vi "get_some_points.vi"(0 "Override":T3, 2 "Stimulus":T1={"Type"=enum."Off", "Phase"=0.0, "Amplitude"=[0.0, 0.0, 0.0, 0.0, 0.0, 0.0], "Injection point"=enum."Total pose", "Closed loop"=TRUE, "Offset"=[0.0, 0.0, 0.0, 0.0, 0.0, 0.0], "Tip -> world"=FALSE, "Frequency"=0.0, "Length"=0.0} {"Length" min=0.0 max=100.0 step=100.0 format="%#_4p"; "Frequency" min=0.0 step=100.0 format="%#_4g"; "Offset" format="%#_3p"; "Amplitude" format="%#_3p"; "Phase" min=-180.0 max=360.0 step=100.0 format="%#.2f"}, 3 "Trace length":dbl=1.0, 5 "Axis names":string[](array[string])=["X", "Y", "Z", "Rx", "Ry", "Rz"], 7 "Sequence":dbl[][](array[numeric]), 11 "error in":errorcluster, 12 "Position mode":enum16{"Absolute axis", "Relative axis", "Pose"}(ring), 14 "Decimate":i32=-1) -> (6 "Decimated trace":sgl[][][][](array[numeric]) format="%#_5g", 15 "error out":errorcluster)   [LabVIEW 2013]
uses:
  ui_override_opts.ctl
  stimulus.ctl
  injection_point.ctl
panel:
  # "This VI uses the motion interface to move the stage to a sequence of points.  At each point it triggers a trace cycle and captures the trace data.  Use with ui_override.vi and single_trigger_setup.vi."
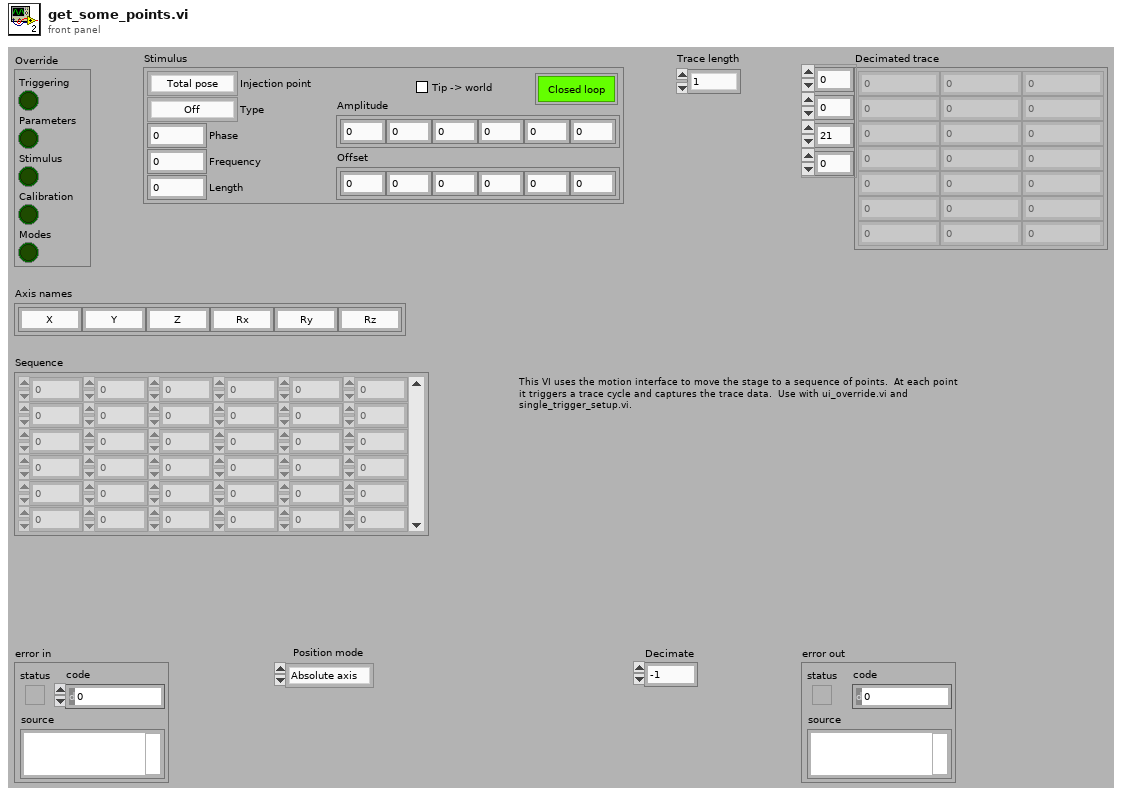
[diagram p1: front panel]
types:
  T1 = typedef "stimulus.ctl" = cluster{"Type":enum16{"Off", "Step", "Sine", "Triangle", "Arbitrary"}, "Phase":dbl, "Amplitude":sgl[], "Injection point":T2, "Closed loop":bool, "Offset":sgl[], "Tip -> world":bool, "Frequency":dbl, "Length":dbl}
  T2 = typedef "injection_point.ctl" = enum16{"Total pose", "V limiter", "Goal ", "Link position", "KF link position", "Inverse kin", "Link goal", "Link error", "Controller", "Output", "Drive", "Light"}
  T3 = typedef "ui_override_opts.ctl" = cluster{"Triggering":bool, "Parameters":bool, "Stimulus":bool, "Calibration":bool, "Modes":bool}
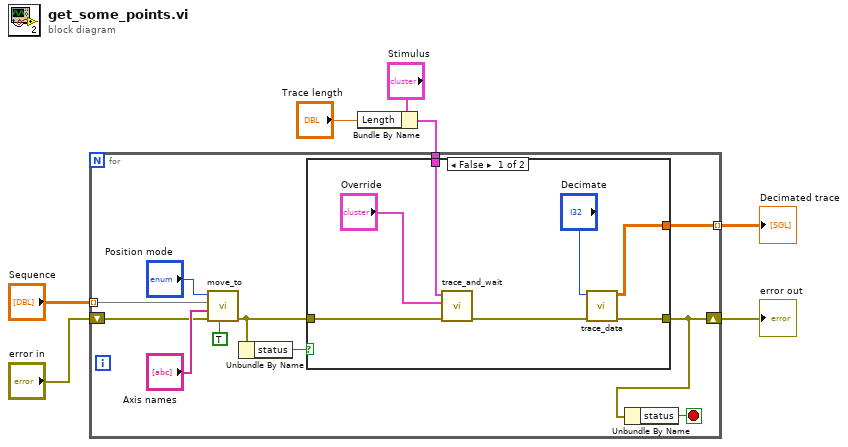
[diagram p0: block diagram]
diagram:
  n1 = Bundle By Name(cluster="Stimulus", "Length"="Trace length") -> (w3:T1)
  n2 = for {
    tunnel: "Sequence" -> [w17] mode=indexing
    shift-right: [w9] -> w6
    shift-left: "error in" -> [w14]
    tunnel: w3 -> [w13]
    tunnel: [w12] -> w1 mode=indexing
    stop <- w8 stop-if-true
    n3 = call "move_to.vi"("Wait until done"=TRUE, "Error in"=w14, "Axis names"="Axis names", "Axis positions"=w17, "Mode"="Position mode") -> ("Error out"=w11:errorcluster)  [unwired: 6 in]
    n4 = Unbundle By Name(w11) -> ("status"=w10:bool)
    n5 = case shown="False" w10 {
      tunnel: w11 -> [w25 w26]
      tunnel: [w21 w26] -> w9
      tunnel: w13 -> [w20 _]
      tunnel: [w19 _] -> w12
      frame False {
        n6 = call "trace_and_wait.vi"("error in"=w25, "Override"="Override", "Stimulus"=w20) -> ("error out"=w23:errorcluster)  [unwired: 8 in]
        n7 = call "trace_data.vi"("error in"=w23, "Decimate"="Decimate") -> ("error out"=w21:errorcluster, "Decimated trace"=w19:sgl[][][])  [unwired: 7 in, 1 out]
      }
      frame True {
      }
    }
    n8 = Unbundle By Name(w9) -> ("status"=w8:bool)
  }
  "error out" <- w6
  "Decimated trace" <- w1
